vi "SFP Get Device Info from Task.vi"(8 "error in":errorcluster, 11 "task":refnum<k21>) -> (0 "error out":errorcluster, 1 "status info out":variant, 3 "device info out":T1 {"Device Info"."Serial Number" format="%x"})   [LabVIEW 2017]
uses:
  <vilib>/addons/Sound and Vibration/svt_DAQmx/subVIs/SFP DAQmx Device Info.ctl
  <resource>/objmgr/daqmx.rc
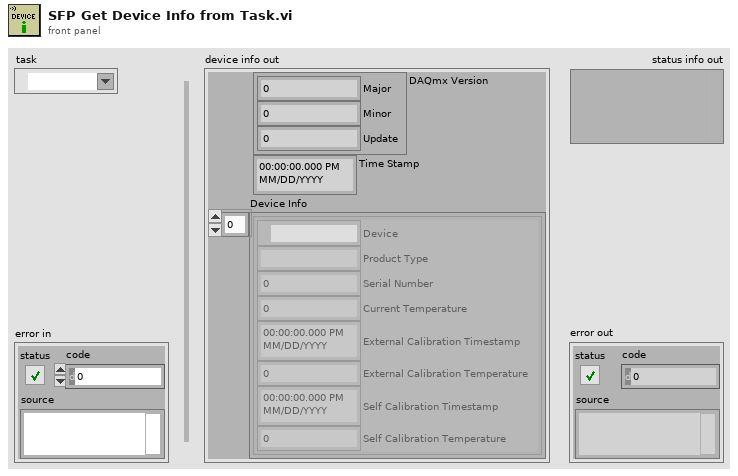
[diagram p1: front panel]
types:
  T1 = typedef "SFP DAQmx Device Info.ctl" = cluster{"DAQmx Version":cluster{"Major":u32, "Minor":u32, "Update":u32}, "Time Stamp":timestamp, "Device Info":cluster{"Device":tag, "Product Type":string, "Serial Number":u32, "Current Temperature":dbl, "External Calibration Timestamp":timestamp, "External Calibration Temperature":dbl, "Self Calibration Timestamp":timestamp, "Self Calibration Temperature":dbl}[]}
  T2 = cluster{"Device":tag, "Product Type":string, "Serial Number":u32, "Current Temperature":dbl, "External Calibration Timestamp":timestamp, "External Calibration Temperature":dbl, "Self Calibration Timestamp":timestamp, "Self Calibration Temperature":dbl}[]
  T3 = cluster{"Device":tag, "Product Type":string, "Serial Number":u32, "Current Temperature":dbl, "External Calibration Timestamp":timestamp, "External Calibration Temperature":dbl, "Self Calibration Timestamp":timestamp, "Self Calibration Temperature":dbl}
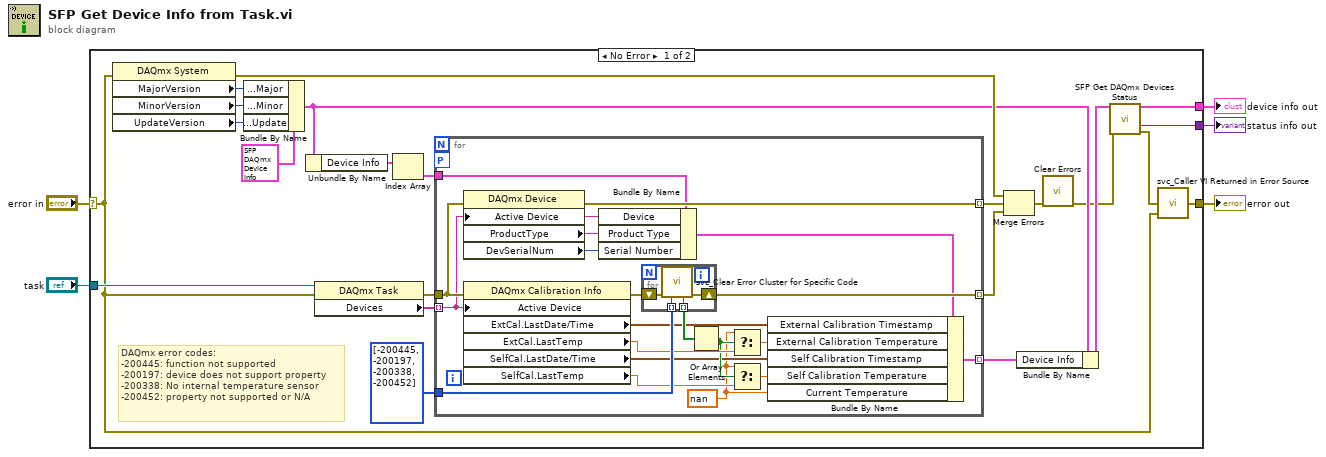
[diagram p0: block diagram]
diagram:
  n1 = case shown="No Error" "error in" {
    selector: "error in" -> [w20 w53]
    tunnel: "task" -> [w27 _]
    tunnel: [w9 _] -> w2
    tunnel: [w19 w53] -> w3
    tunnel: [w6 _] -> w1
    frame No Error {
      # "DAQmx error codes:\n-200445: function not supported\n-200197: device does not support property\n-200338: No internal temperature sensor\n-200452: property not supported or N/A"
      n2 = property class="DAQmx System"(error in=w20) -> (error out=w24:errorcluster, "MajorVersion"=w15:u32, "MinorVersion"=w14:u32, "UpdateVersion"=w13:u32)  [unwired: 1 in, 1 out]
      n3 = Bundle By Name(cluster=T1 {"DAQmx Version"={"Major"=0, "Minor"=0, "Update"=0}, "Time Stamp"=timestamp(0 s since 1904-01-01), "Device Info"=[]}, "DAQmx Version.Major"=w15, "DAQmx Version.Minor"=w14, "DAQmx Version.Update"=w13) -> (w11:T1)
      n4 = Unbundle By Name(w11) -> ("Device Info"=w16:T2)
      n5 = property class="DAQmx Task"(reference=w27, error in=w20) -> (error out=w26:errorcluster, "Devices"=w28:tag[])  [unwired: 1 out]
      n6 = Index Array(array=w16) -> (element=w17:T3)  [unwired: 1 in]
      n7 = for {
        tunnel: w28 -> [w34] mode=indexing
        tunnel: [w30] -> w25 mode=indexing
        workers-P: _ -> [_]
        tunnel: w26 -> [w48]
        tunnel: [w47] -> w23 mode=indexing
        tunnel: [w42] -> w22 mode=indexing
        tunnel: i32[] [-200445, -200197, -200338, -200452] ("DAQmx error codes:") -> [w45]
        tunnel: w17 -> [w35]
        w29 = nan ("t")
        n8 = property class="DAQmx Device"(error in=w48, "Active Device"=w34) -> (error out=w47:errorcluster, "ProductType"=w33:string, "DevSerialNum"=w32:u32)  [unwired: 1 in, 1 out]
        n9 = property class="DAQmx Calibration Info"(error in=w48, "Active Device"=w34) -> (error out=w46:errorcluster, "ExtCal.LastDate/Time"=w36:timestamp, "ExtCal.LastTemp"=w44:dbl, "SelfCal.LastDate/Time"=w38:timestamp, "SelfCal.LastTemp"=w43:dbl)  [unwired: 1 in, 1 out]
        n10 = Bundle By Name(cluster=w35, "Device"=w34, "Product Type"=w33, "Serial Number"=w32) -> (w31:T3)
        n11 = for {
          tunnel: w45 -> [w51] mode=indexing
          tunnel: [w49] -> w40 mode=indexing
          shift-right: [w50] -> w42
          shift-left: w46 -> [w52]
          n12 = call <vilib>:"svc_Clear Error Cluster for Specific Code.vi"("error in (no error)"=w52, "code"=w51) -> ("error cleared"=w49:bool, "error out"=w50:errorcluster)  [unwired: 12 in]
        }
        n13 = Or Array Elements(Boolean array=w40) -> (logical OR=w41:bool)
        n14 = Select(t=w29, s=w41, f=w44) -> (s? t:f=w37:dbl)
        n15 = Select(t=w29, s=w41, f=w43) -> (s? t:f=w39:dbl)
        n16 = Bundle By Name(cluster=w31, "External Calibration Timestamp"=w36, "External Calibration Temperature"=w37, "Self Calibration Timestamp"=w38, "Self Calibration Temperature"=w39, "Current Temperature"=w29) -> (w30:T3)
      }
      n17 = Merge Errors(w24, w23, w22) -> (w18:errorcluster)
      n18 = Bundle By Name(cluster=w11, "Device Info"=w25) -> (w10:T1)
      n19 = call <vilib>:"Clear Errors.vi"("error in (no error)"=w18) -> ("error out"=w8:errorcluster)  [unwired: 5 in, 1 out]
      n20 = call <vilib>:"SFP Get DAQmx Devices Status.vi"("device info"=w10, "error in"=w8) -> ("device info"=w9:T1, "status info out"=w6:variant, "error out"=w7:errorcluster)  [unwired: 11 in]
      n21 = call <vilib>:"svc_Caller VI Returned in Error Source.vi"("warning input to caller"=w20, "error in (no error)"=w7) -> ("error out"=w19:errorcluster)  [unwired: 3 in]
    }
    frame Error {
    }
  }
  "device info out" <- w2
  "error out" <- w3
  "status info out" <- w1
